vi "Broadcast Batch Messages.vi"(8 "error in (no error)":errorcluster, 10 "Messages In":refnum<class "Message.lvclass">[](array[class]), 11 "Messenger in":refnum<class "Tree-ArrayLocation Queue Messenger.lvclass">) -> (0 "error out":errorcluster, 3 "Messenger out":refnum<class "Tree-ArrayLocation Queue Messenger.lvclass">)   [LabVIEW 2019, in "Tree-ArrayLocation Queue Messenger.lvclass"]
uses:
  Tree-ArrayLocation Queue Messenger.lvclass
  C:/Users/iio/Desktop/NTHU Brain Center/General Purpose/Classes/Ancestor/Messenger/Messenger Composite/Messenger Composite.lvclass
  Ancestor Class/Message/Message.lvclass
  Tree-ArrayLocation Queue Messenger.lvclass/Tree-ArrayLocation Queue Messenger.ctl
  Ancestor Class/Messenger/Messenger Composite/Messenger Composite.lvclass/Messenger Composite.ctl
  Ancestor Class/Messenger/Messenger Composite/Public Data/Read Nodes.vi
  Ancestor Class/Messenger/Messenger/Messenger.lvclass
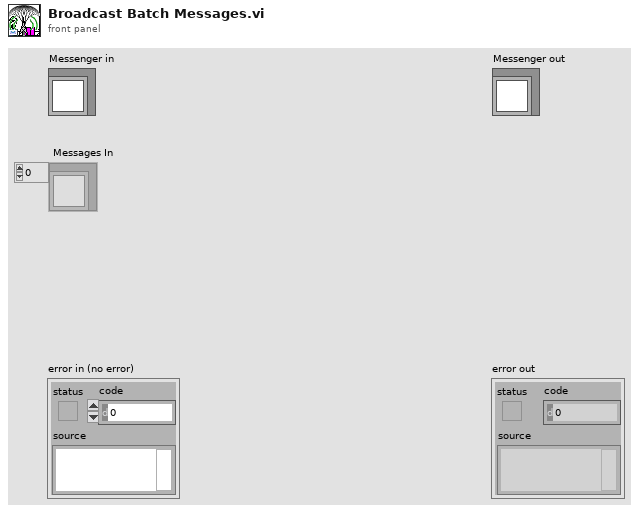
[diagram p1: front panel]
types:
  T1 = typedef "Message Queue.ctl" = refnum<queue>
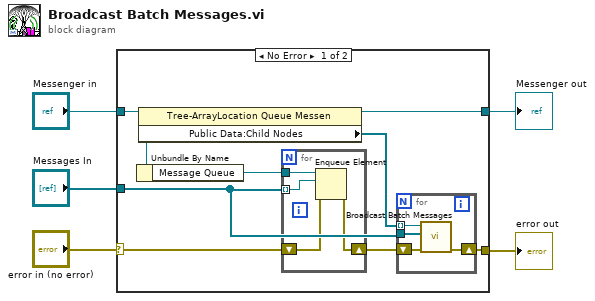
[diagram p0: block diagram]
diagram:
  n1 = case shown="No Error" "error in (no error)" {
    selector: "error in (no error)" -> [w12 w23]
    tunnel: [w10 w23] -> w4
    tunnel: [w6 w22] -> w3
    tunnel: "Messenger in" -> [w8 w22]
    tunnel: "Messages In" -> [w9 _]
    frame No Error {
      n2 = Unbundle By Name(w8) -> ("Message Queue"=w13:T1)
      n3 = property class="Tree-ArrayLocation Queue Messen"(reference=w8) -> (reference out=w6:refnum<class "Tree-ArrayLocation Queue Messenger.lvclass">, "Public Data:Child Nodes"=w7:refnum<class "Messenger.lvclass">[])  [unwired: 1 in, 1 out]
      n4 = for {
        tunnel: w13 -> [w21]
        tunnel: w9 -> [w20] mode=indexing
        shift-right: [w18] -> w11
        shift-left: w12 -> [w19]
        n5 = Enqueue Element(queue=w21, element=w20, error in (no error)=w19) -> (error out=w18:errorcluster)  [unwired: 1 in, 2 out]
      }
      n6 = for {
        shift-right: [w14] -> w10
        shift-left: w11 -> [w15]
        tunnel: w7 -> [w17] mode=indexing
        tunnel: w9 -> [w16]
        n7 = call-dynamic "Broadcast Batch Messages.vi"("error in (no error)"=w15, "Messages In"=w16, "Messenger in"=w17) -> ("error out"=w14:errorcluster)  [unwired: 7 in, 1 out]
      }
    }
    frame Error {
    }
  }
  "error out" <- w4
  "Messenger out" <- w3
